vi "MoveData.vi"(8 "error in (no error)":errorcluster, 11 "Package Builder in":refnum<class "Package Builder.lvclass">) -> (0 "error out":errorcluster, 3 "Package Builder out":refnum<class "Package Builder.lvclass">)   [LabVIEW 2020, in "Package Builder.lvclass"]
uses:
  Package Builder.lvclass
  Package Builder.lvclass/Package Builder.ctl
panel:
  out "Destination Folder":path
  out "Source Folder":path
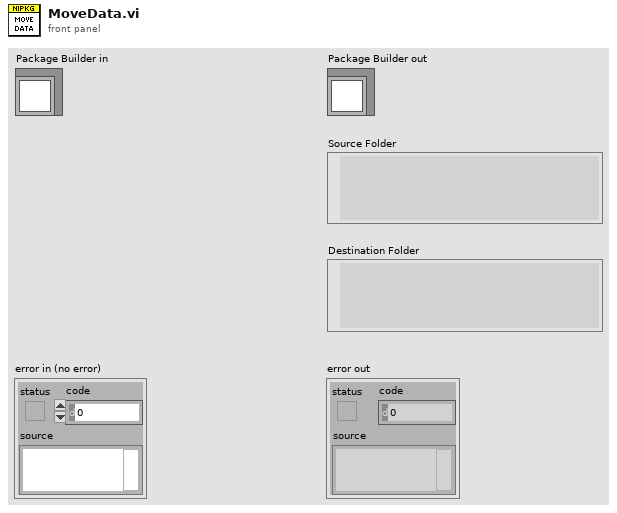
[diagram p1: front panel]
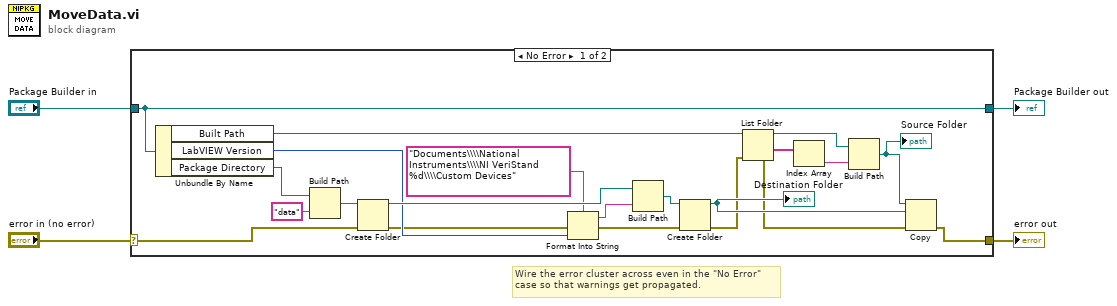
[diagram p0: block diagram]
diagram:
  # "Wire the error cluster across even in the \"No Error\"\ncase so that warnings get propagated."
  n1 = case shown="No Error" "error in (no error)" {
    selector: "error in (no error)" -> [w18 w27]
    tunnel: [w10 w27] -> w3
    tunnel: [w20 w26] -> w1
    tunnel: "Package Builder in" -> [w20 w26]
    frame No Error {
      n2 = Unbundle By Name(w20) -> ("Built Path"=w14:path, "LabVIEW Version"=w6:u32, "Package Directory"=w19:path)
      n3 = Build Path(base path=w19, name or relative path="data" ("time format string (%c)")) -> (appended path=w25:path)
      n4 = Create Folder(path (use dialog)=w25, error in=w18) -> (created path=w23:path, error out=w5:errorcluster)  [unwired: 1 in, 1 out]
      n5 = Format Into String(format string="Documents\\\\National Instruments\\\\NI VeriStand %d\\\\Custom Devices" ("time format string (%c)"), error in=w5, w6) -> (resulting string=w8:string, error out=w7:errorcluster)  [unwired: 1 in]
      n6 = Build Path(base path=w23, name or relative path=w8) -> (appended path=w22:path)
      n7 = Create Folder(path (use dialog)=w22, error in=w7) -> (created path=w21:path, error out=w17:errorcluster)  [unwired: 1 in, 1 out]
      "Destination Folder" <- w21
      n8 = List Folder(path=w14, error in=w17) -> (path out=w11:path, folder names=w15:string[], error out=w16:errorcluster)  [unwired: 2 in, 1 out]
      n9 = Index Array(array=w15) -> (element=w13:string)  [unwired: 1 in]
      n10 = Build Path(base path=w11, name or relative path=w13) -> (appended path=w12:path)
      "Source Folder" <- w12
      n11 = Copy(8:w16, 10:w21, 11:w12) -> (0:w10:errorcluster)  [unwired: 2 in, 2 out]
    }
    frame Error {
    }
  }
  "error out" <- w3
  "Package Builder out" <- w1
